vi "Window-Coordinates window exit dialogue.vi"(11 "Input cluster":T1={"Caption-Right button"="", "Caption-Left button"="", "Message to display"="", "Delay before close"=0, "Window Colour"=16448250, "Cancel button disabled?"=enum."Enabled"}) -> (3 "Left Button (Cancel)":bool)   [LabVIEW 2013]
uses:
  Global Variables/General Globals.vi
panel:
  in  "Left Button (Cancel)":bool
  in  "Right Button":bool
  out "Message display":string
  out "Window Colour":u32(colorbox)=16448250
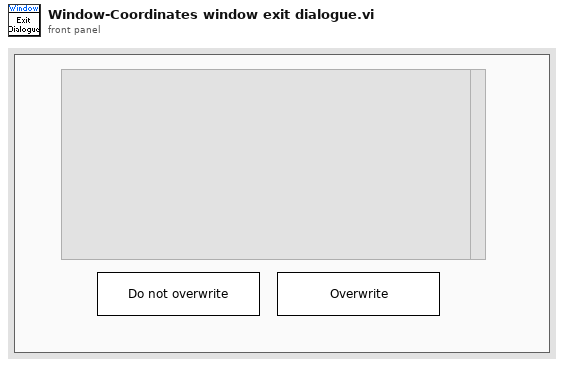
[diagram p1: front panel]
types:
  T1 = cluster{"Caption-Right button":string, "Caption-Left button":string, "Message to display":string, "Delay before close":u32, "Window Colour":u32, "Cancel button disabled?":enum8{"Enabled", "Disabled", "Disabled and Grayed Out"}}
  T2 = enum8{"Enabled", "Disabled", "Disabled and Grayed Out"}
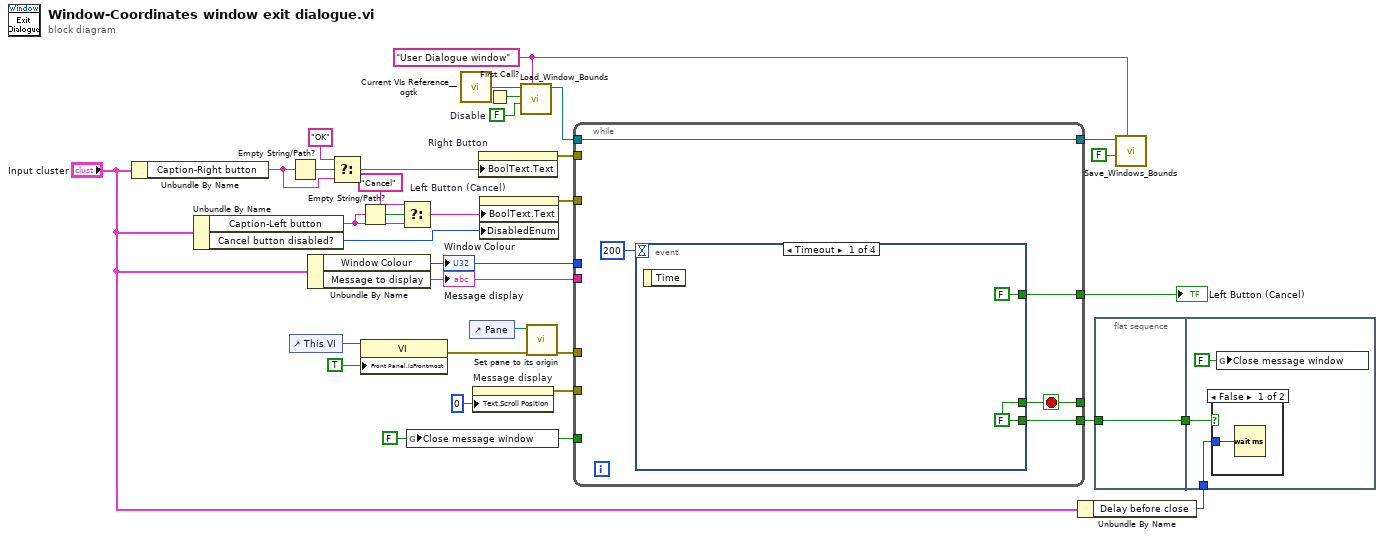
[diagram p0: block diagram]
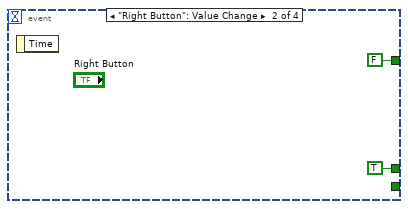
[diagram p3: hidden frame]
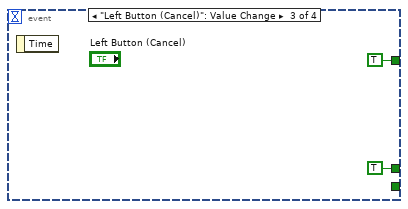
[diagram p4: hidden frame]
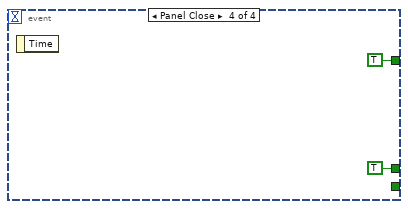
[diagram p5: hidden frame]
diagram:
  w4 = FALSE ("Close message window")
  w11 = FALSE  # Disable
  w10 = "User Dialogue window" ("Window Name (i.e. Key)")
  n1 = Unbundle By Name("Input cluster") -> ("Caption-Right button"=w20:string)
  n2 = Unbundle By Name("Input cluster") -> ("Caption-Left button"=w19:string, "Cancel button disabled?"=w14:T2)
  n3 = Empty String/Path?(string/path=w20) -> (empty?=w28:bool)
  n4 = control-ref of="This VI"() -> (w2:refnum<vi>)
  n5 = Unbundle By Name("Input cluster") -> ("Window Colour"=w15:u32, "Message to display"=w18:string)
  "Window Colour" <- w15
  "Message display" <- w18
  n6 = Select(t="OK", s=w28, f=w20) -> (s? t:f=w26:string)
  n7 = Empty String/Path?(string/path=w19) -> (empty?=w24:bool)
  n8 = property on="Property Node" class="VI"(reference=w2, "Front Panel.IsFrontmost"=TRUE ("Front Panel Window:Is Frontmost")) -> (error out=w1:errorcluster)  [unwired: 1 in, 1 out]
  n9 = Select(t="Cancel", s=w24, f=w19) -> (s? t:f=w23:string)
  n10 = global write "General Globals.vi" "Close message window"(w4) -> ()
  n11 = call "Current VIs Reference__ogtk.vi"() -> ("Current VI's reference"=w13:refnum<vi>)  [unwired: 5 in]
  n12 = control-ref of="Pane"() -> (w33:refnum<vi>)
  n13 = property on="Message display" class="Str"("Text.Scroll Position"=u32 0) -> (error out=w5:errorcluster)  [unwired: 2 in, 1 out]
  n14 = property on="Right Button" class="Bool"("BoolText.Text"=w26) -> (error out=w29:errorcluster)  [unwired: 2 in, 1 out]
  n15 = property on="Left Button (Cancel)" class="Bool"("BoolText.Text"=w23, "DisabledEnum"=w14) -> (error out=w30:errorcluster)  [unwired: 2 in, 1 out]
  n16 = First Call?() -> (First Call?: T/F=w12:bool)
  n17 = call "Load_Window_Bounds.vi"("Window Name (i.e. Key)"=w10, "Disable"=w11, "First Call"=w12, "Window VI's Ref"=w13) -> ("reference out"=w7:refnum<vi>)  [unwired: 4 in, 3 out]
  n18 = call "Set pane to its origin.vi"("error in (no error)"=w1, "Pane Reference"=w33) -> ("error out (no error)"=w32:errorcluster)  [unwired: 8 in, 1 out]
  n19 = while {
    tunnel: w18 -> [_]
    tunnel: w32 -> [_]
    tunnel: w15 -> [_]
    tunnel: [w38] -> _
    tunnel: [w36] -> w31
    tunnel: w30 -> [_]
    tunnel: w29 -> [_]
    tunnel: [w35] -> w22
    tunnel: w7 -> [w34]
    tunnel: [w34] -> w8
    tunnel: w5 -> [_]
    tunnel: w4 -> [_]
    stop <- w38 stop-if-true
    n20 = event shown="[0] Timeout" {
      selector: _ -> [_ _ _ _]
      dyn-events: _ -> [_ _ _ _]
      timeout: 200 -> [_ _ _ _]
      tunnel: [w39 TRUE TRUE TRUE] -> w38
      tunnel: [FALSE ("Cancel") FALSE ("Cancel") TRUE ("Cancel") TRUE ("Cancel")] -> w36
      tunnel: [w39 _ _ _] -> w35
      event Timeout {
        w39 = FALSE
        n21 = event-data() -> ()  [unwired: 1 in, 1 out]
      }
      event "Right Button": Value Change {
        n22 = event-data() -> ()  [unwired: 1 in, 1 out]
      }
      event "Left Button (Cancel)": Value Change {
        n23 = event-data() -> ()  [unwired: 1 in, 1 out]
      }
      event Panel Close {
        n24 = event-data() -> ()  [unwired: 1 in, 1 out]
      }
    }
  }
  "Left Button (Cancel)" <- w31
  n25 = Unbundle By Name("Input cluster") -> ("Delay before close"=w17:u32)
  n26 = flat-sequence {
    tunnel: [w47] -> w21
    tunnel: w22 -> [w47]
    tunnel: w17 -> [w50]
    tunnel: w21 -> [w49]
    frame #0 {
    }
    frame #1 {
      n27 = case shown="False" w49 {
        tunnel: w50 -> [w51 _]
        frame False {
          n28 = Wait (ms)(milliseconds to wait=w51) -> ()  [unwired: 1 out]
        }
        frame True {
        }
      }
      n29 = global write "General Globals.vi" "Close message window"(FALSE ("Close message window")) -> ()
    }
  }
  n30 = call "Save_Windows_Bounds.vi"("Window Name (i.e. Key)"=w10, "Front Panel Window:Open"=FALSE, "Window VI's Ref"=w8) -> ()  [unwired: 8 in, 1 out]
